vi "Get SMO Port.vi"(8 "error in (no error)":errorcluster, 11 "Instrument.TC in":refnum<class "Instrument.TC.lvclass">) -> (0 "error out":errorcluster, 2 "Port":u16, 3 "Instrument.TC out":refnum<class "Instrument.TC.lvclass">)   [LabVIEW 2019, in "Instrument.TC.lvclass"]
uses:
  Instrument.TC.lvclass
  <userlib>/LevyLab/Instrument Framework/Instrument Types/Cryostat/Instrument.Cryostat.lvclass
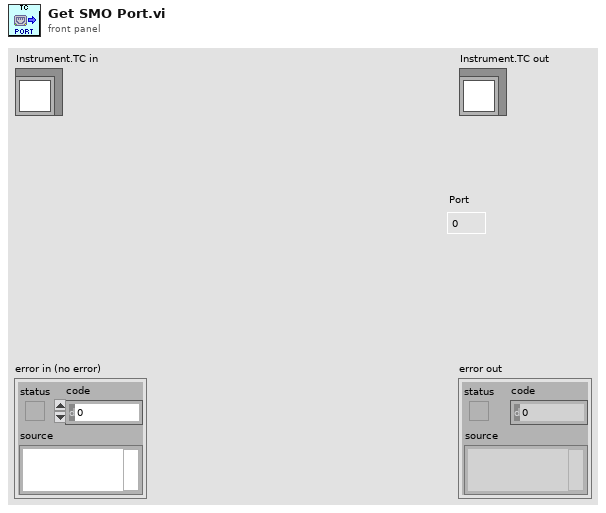
[diagram p1: front panel]
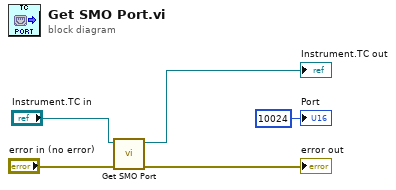
[diagram p0: block diagram]
diagram:
  n1 = call-parent "Get SMO Port.vi"("error in (no error)"="error in (no error)", "Instrument in"="Instrument.TC in") -> ("error out"=→"error out":errorcluster, "Instrument out"=→"Instrument.TC out":refnum<class "Instrument.TC.lvclass">)  [unwired: 7 in, 1 out]
  "Port" <- u16 10024 ("Port")
